vi "Global 1.vi"() -> ()   [LabVIEW 2015]
panel:
  out "error":dbl
  out "last encoder":dbl
  out "encoder":dbl
  out "current":dbl
  out "Timer":dbl
  out "Motor speed":dbl
  out "position":dbl
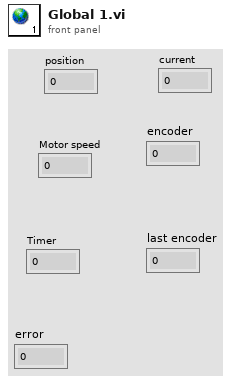
[diagram p1: front panel]
diagram:
